vi "Get Sphere S Aand Vol.vi"(3 "sa":dbl, 4 "vol":dbl, 5 "radius":dbl, 6 "path in":path) -> (0 "sa out":dbl, 1 "vol out":dbl, 2 "function return":i32)   [LabVIEW 2018]
doc: "extern \"C\" __declspec(dllexport) int GetSphereSAandVol(double radius, double* sa, double* vol);"
panel:
  out "appended path":path
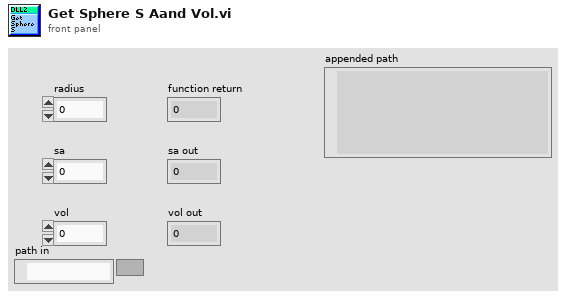
[diagram p1: front panel]
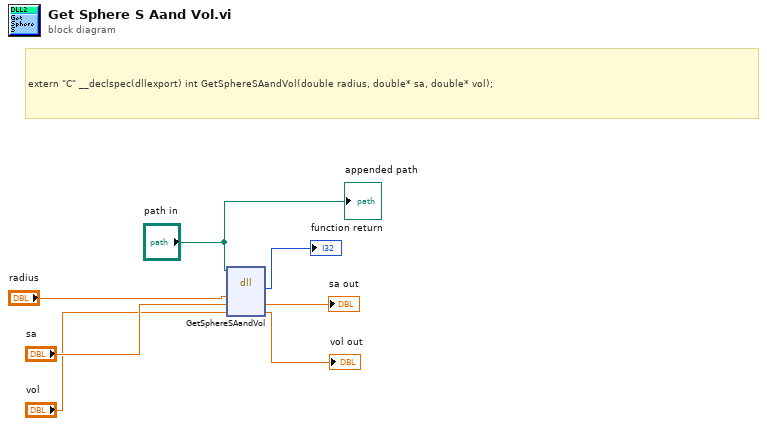
[diagram p0: block diagram]
diagram:
  # "extern \"C\" __declspec(dllexport) int GetSphereSAandVol(double radius, double* sa, double* vol);"
  n1 = dll-call lib="C:/Users/celit/Documents/GitHub/Labview_Python_DLL_Call/vs/Debug/Labview_to_DLL.dll" fn="GetSphereSAandVol"(path in="path in", "radius"="radius", "sa"="sa", "vol"="vol") -> ("return type"=→"function return":i32, "sa"=→"sa out":dbl, "vol"=→"vol out":dbl)  [unwired: 3 in, 2 out]
  "appended path" <- "path in"
